vi "WriteFileIV.vi"(8 "error in":errorcluster, 11 "File Name":string) -> (0 "error out":errorcluster, 3 "appended path":path)   [LabVIEW 2020]
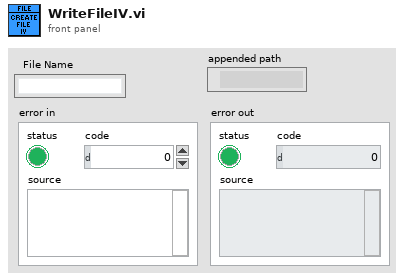
[diagram p1: front panel]
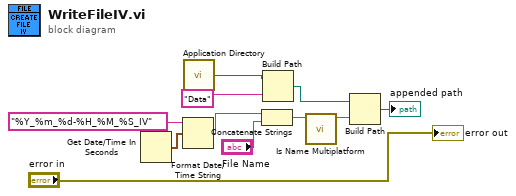
[diagram p0: block diagram]
diagram:
  n1 = Get Date/Time In Seconds() -> (seconds since 1Jan1904=w3:timestamp)
  n2 = Format Date/Time String(time format string (%c)="%Y_%m_%d-%H_%M_%S_IV", seconds (now)=w3) -> (date/time string=w10:string)  [unwired: 1 in]
  n3 = call <vilib>:"Application Directory.vi"() -> ("Application Directory"=w8:path)
  n4 = Concatenate Strings(w10, "File Name") -> (w5:string)
  n5 = Build Path(base path=w8, name or relative path="Data") -> (appended path=w7:path)
  n6 = call <vilib>:"Is Name Multiplatform.vi"("filename"=w5) -> ("suggested filename"=w4:string)  [unwired: 6 in, 4 out]
  n7 = Build Path(base path=w7, name or relative path=w4) -> (appended path=→"appended path":path)
  "error out" <- "error in"
